vi "Set RPM.vi"(2 "EncoderDevRef":T1={"DevStatus"={"status"=FALSE, "code"=0, "source"=""}, "EncoderIndex"=enum."Invalid", "CounterIndex"=enum."Ctr 1", "DistancePerCount"=2.0, "Decoding Type"=enum."4x"}, 3 "Height":dbl, 4 "Angle":dbl, 5 "Distance":dbl) -> (0 "Ready to shoot":bool, 1 "Thrower Voltage":dbl)   [LabVIEW 2011]
uses:
  <vilib>/Rock Robotics/SystemInterfaces/Encoder/FPGA_EncoderIdx.ctl
  <vilib>/Rock Robotics/WPI/Encoder/WPI_EncoderType.ctl
  <vilib>/Rock Robotics/SystemInterfaces/Counter/FPGA_CounterCtrSystemIndex.ctl
  <vilib>/Rock Robotics/WPI/Encoder/WPI_EncoderDevRef.ctl
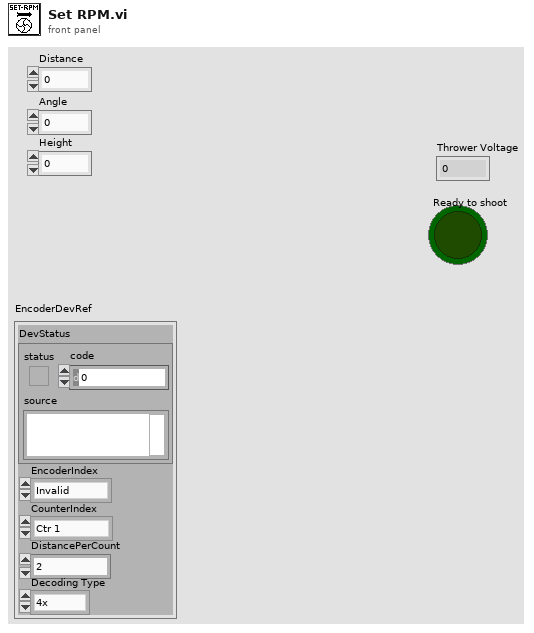
[diagram p1: front panel]
types:
  T1 = typedef "WPI_EncoderDevRef.ctl" = cluster{"DevStatus":errorcluster, "EncoderIndex":T2, "CounterIndex":T3, "DistancePerCount":dbl, "Decoding Type":T4}
  T2 = typedef "FPGA_EncoderIdx.ctl" = enum8{"Enc 0", "Enc 1", "Enc 2", "Enc 3", "Invalid"}
  T3 = typedef "FPGA_CounterCtrSystemIndex.ctl" = enum8{"Ctr 0", "Ctr 1", "Ctr 2", "Ctr 3", "Ctr 4", "Ctr 5", "Ctr 6", "Ctr 7", "Invalid"}
  T4 = typedef "WPI_EncoderType.ctl" = enum16{"1x", "2x", "4x"}
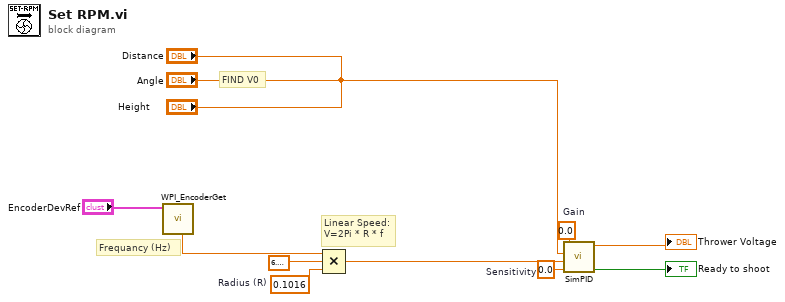
[diagram p0: block diagram]
diagram:
  w5 = 0.0  # Gain
  w6 = 0.0  # Sensitivity
  w8 = 0.1016  # Radius (R)
  # "FIND V0"
  # "Linear Speed:\nV=2Pi * R * f"
  # "Frequancy (Hz)"
  n1 = call <vilib>:"WPI_EncoderGet.vi"("EncoderDevRef"="EncoderDevRef") -> ("Rate"=w10:dbl)  [unwired: 5 in, 5 out]
  n2 = Compound Arithmetic op=MULTIPLY(w10, 6.283185307179586, w8) -> (w7:dbl)
  n3 = call "SimPID.vi"("Range"=w6, "Position"=w7, "Set Point"="Angle", "Gain"=w5) -> ("On Target"=→"Ready to shoot":bool, "result"=→"Thrower Voltage":dbl)  [unwired: 5 in]
  "Distance" <- "Angle"
  "Height" <- "Angle"
